vi "PercentageToRGB.vi"(10 "percentage":dbl(slide) scale=0.0..1.0) -> (2 "rgb":u32)   [LabVIEW 2017]
panel:
  out "Array":dbl[](array[numeric])
  out "log(x)":dbl[](array[numeric])
  out "Color Box":u32(colorbox)
  in  "type":enum16{"Temperature", "Greyscale", "Heatmap"}(ring)=enum."Heatmap"
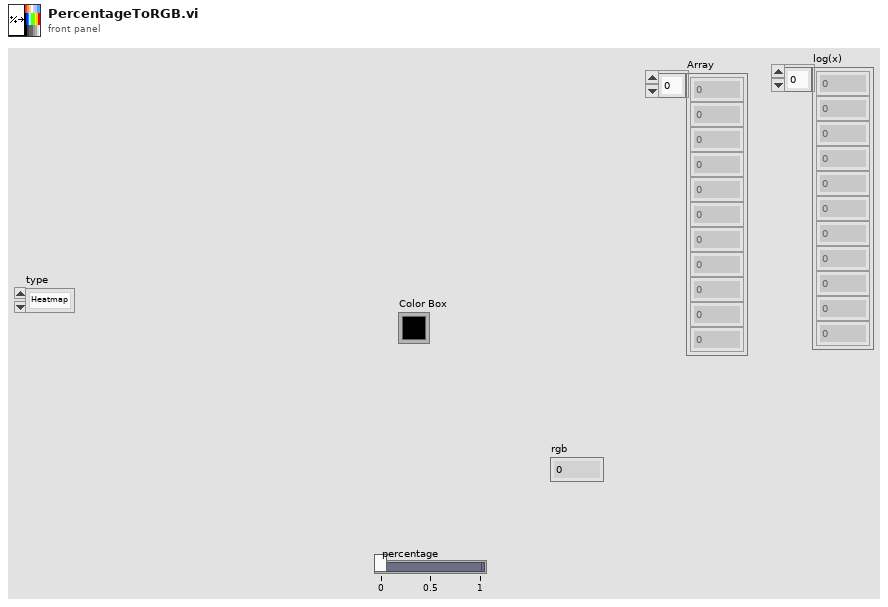
[diagram p1: front panel]
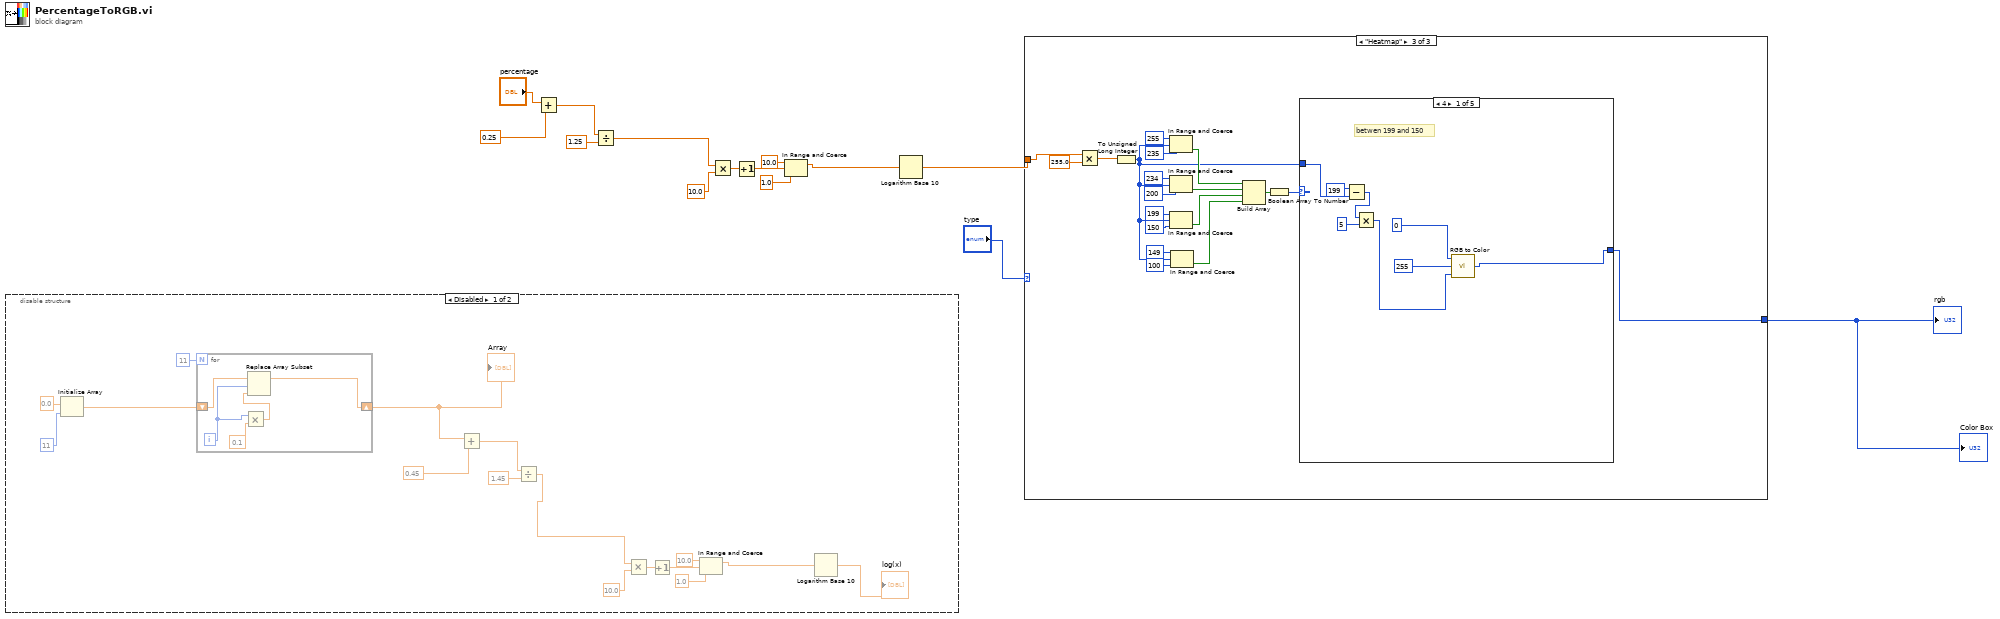
[diagram p0: block diagram]
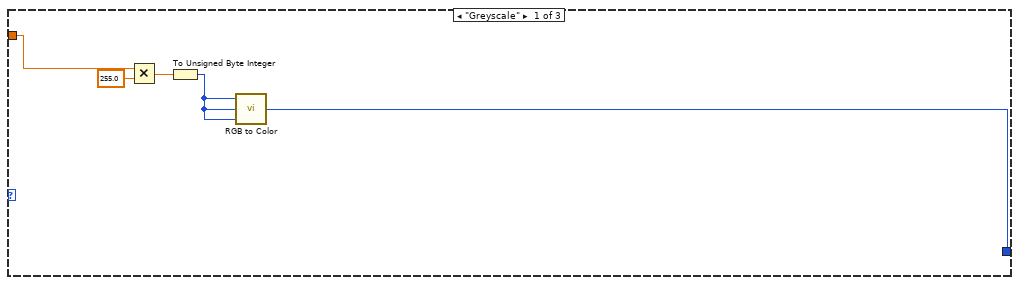
[diagram p3: hidden frame]
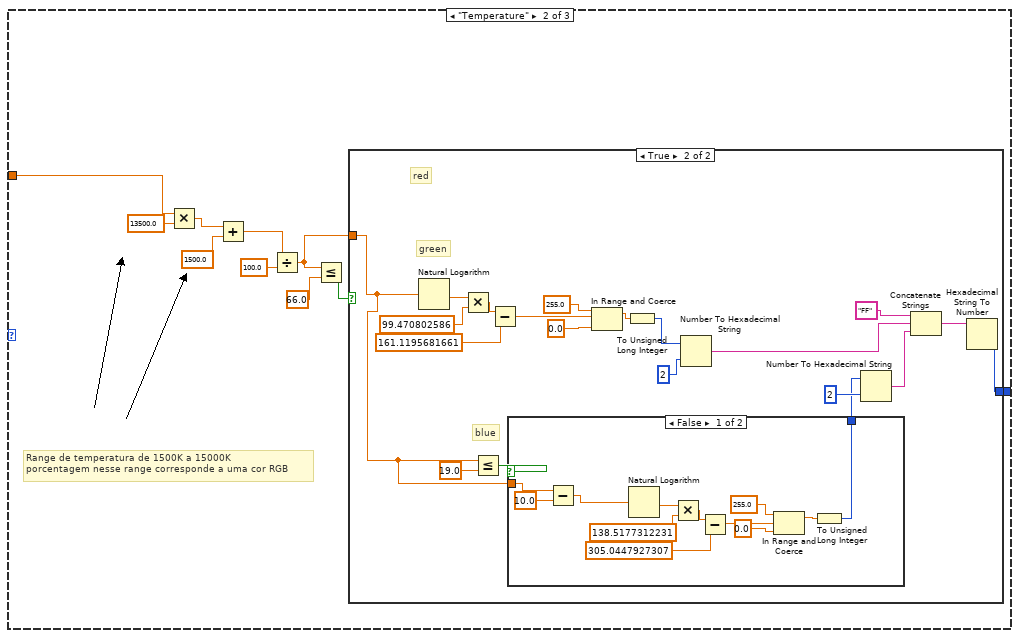
[diagram p4: hidden frame]
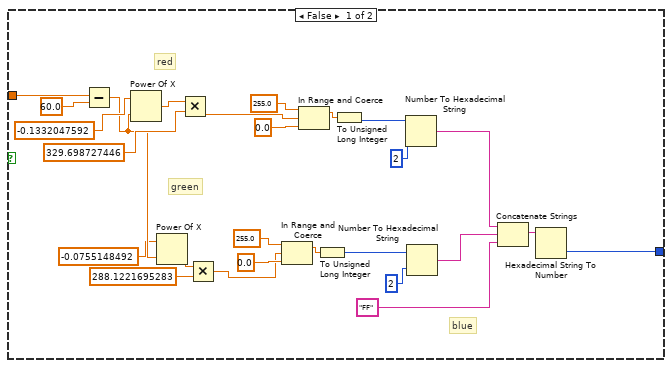
[diagram p5: hidden frame]
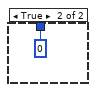
[diagram p6: hidden frame]
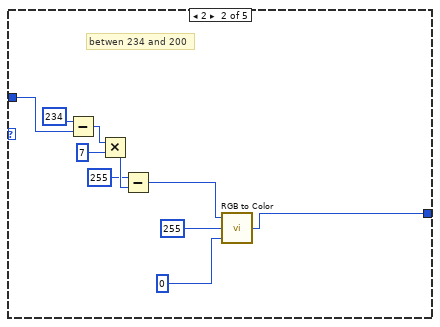
[diagram p7: hidden frame]
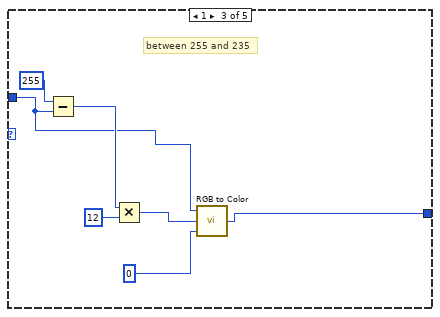
[diagram p8: hidden frame]
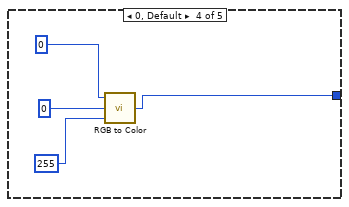
[diagram p9: hidden frame]
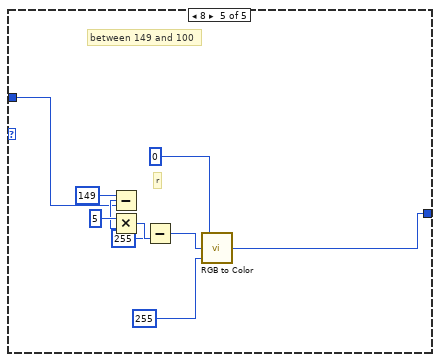
[diagram p10: hidden frame]
diagram:
  n1 = disable-structure shown="Disabled" {
    frame Disabled {
      n2 = Initialize Array(0.0 ("element"), 11 ("dimension size")) -> (w29:dbl[])
      n3 = for {
        N: 11 -> [_]
        shift-right: [w31] -> w16
        shift-left: w29 -> [w35]
        i -> [w33]
        n4 = Multiply(x=w33, y=0.1) -> (x*y=w34:dbl)
        n5 = Replace Array Subset(array=w35, new element=w34, index=w33) -> (w31:dbl[])
      }
      "Array" <- w16
      n6 = Add(x=w16, y=0.45) -> (x+y=w18:dbl[])
      n7 = Divide(x=w18, y=1.45) -> (x/y=w15:dbl[])
      n8 = Multiply(x=w15, y=10.0) -> (x*y=w25:dbl[])
      n9 = Increment(x=w25) -> (x+1=w24:dbl[])
      n10 = In Range and Coerce(upper limit=10.0, x=w24, lower limit=1.0) -> (coerced(x)=w21:dbl[])  [unwired: 1 out]
      n11 = Logarithm Base 10(1:w21) -> (0:→"log(x)":dbl[])
    }
    frame Enabled {
    }
  }
  n12 = Add(x="percentage", y=0.25) -> (x+y=w3:dbl)
  n13 = Divide(x=w3, y=1.25) -> (x/y=w1:dbl)
  n14 = Multiply(x=w1, y=10.0) -> (x*y=w11:dbl)
  n15 = Increment(x=w11) -> (x+1=w9:dbl)
  n16 = In Range and Coerce(upper limit=10.0, x=w9, lower limit=1.0) -> (coerced(x)=w6:dbl)  [unwired: 1 out]
  n17 = Logarithm Base 10(1:w6) -> (0:w10:dbl)
  n18 = case shown="\"Heatmap\"" "type" {
    tunnel: w10 -> [w40 w48 w128]
    tunnel: [w36 w43 w110] -> w13
    frame "Greyscale" {
      n19 = Multiply(x=w40, y=255.0) -> (x*y=w38:dbl)
      n20 = To Unsigned Byte Integer(number=w38) -> (unsigned 8bit integer=w37:u8)
      n21 = call <vilib>:"RGB to Color.vi"("B"=w37, "G"=w37, "R"=w37) -> ("Color"=w36:u32)
    }
    frame "Temperature" {
      # "Range de temperatura de 1500K a 15000K\nporcentagem nesse range corresponde a uma cor RGB"
      n22 = Multiply(x=w48, y=13500.0) -> (x*y=w49:dbl)
      n23 = Add(x=w49, y=1500.0) -> (x+y=w41:dbl)
      n24 = Divide(x=w41, y=100.0) -> (x/y=w44:dbl)
      n25 = Less Or Equal?(x=w44, y=66.0) -> (x <= y?=w45:bool)
      n26 = case shown="True" w45 {
        tunnel: w44 -> [w76 w85]
        tunnel: [w64 w88] -> w43
        frame False {
          # "blue"
          # "green"
          # "red"
          n27 = Subtract(x=w76, y=60.0) -> (x-y=w52:dbl)
          n28 = Power Of X(1:w52, 2:-0.1332047592 ("x")) -> (0:w74:dbl)
          n29 = Power Of X(1:w52, 2:-0.0755148492 ("x")) -> (0:w72:dbl)
          n30 = Multiply(x=w74, y=329.698727446) -> (x*y=w60:dbl)
          n31 = Multiply(x=w72, y=288.1221695283) -> (x*y=w55:dbl)
          n32 = In Range and Coerce(upper limit=255.0, x=w55, lower limit=0.0) -> (coerced(x)=w56:dbl)  [unwired: 1 out]
          n33 = In Range and Coerce(upper limit=255.0, x=w60, lower limit=0.0) -> (coerced(x)=w61:dbl)  [unwired: 1 out]
          n34 = To Unsigned Long Integer(number=w56) -> (unsigned 32bit integer=w54:u32)
          n35 = To Unsigned Long Integer(number=w61) -> (unsigned 32bit integer=w59:u32)
          n36 = Number To Hexadecimal String(1:i16 2 ("width (-)"), 2:w59) -> (0:w68:string)
          n37 = Number To Hexadecimal String(1:i16 2 ("width (-)"), 2:w54) -> (0:w67:string)
          n38 = Concatenate Strings(w68, w67, "FF" ("string")) -> (w65:string)
          n39 = Hexadecimal String To Number(string=w65) -> (number=w64:u32)  [unwired: 2 in, 1 out]
        }
        frame True {
          # "blue"
          # "green"
          # "red"
          n40 = Natural Logarithm(1:w85) -> (0:w95:dbl)
          n41 = Multiply(x=w95, y=99.470802586) -> (x*y=w93:dbl)
          n42 = Less Or Equal?(x=w85, y=19.0) -> (x <= y?=w86:bool)
          n43 = Subtract(x=w93, y=161.1195681661) -> (x-y=w84:dbl)
          n44 = case shown="False" w86 {
            tunnel: w85 -> [w104 _]
            tunnel: [w97 u32 0] -> w78
            frame False {
              n45 = Subtract(x=w104, y=10.0) -> (x-y=w102:dbl)
              n46 = Natural Logarithm(1:w102) -> (0:w108:dbl)
              n47 = Multiply(x=w108, y=138.5177312231) -> (x*y=w106:dbl)
              n48 = Subtract(x=w106, y=305.0447927307) -> (x-y=w98:dbl)
              n49 = In Range and Coerce(upper limit=255.0, x=w98, lower limit=0.0) -> (coerced(x)=w99:dbl)  [unwired: 1 out]
              n50 = To Unsigned Long Integer(number=w99) -> (unsigned 32bit integer=w97:u32)
            }
            frame True {
            }
          }
          n51 = In Range and Coerce(upper limit=255.0, x=w84, lower limit=0.0) -> (coerced(x)=w81:dbl)  [unwired: 1 out]
          n52 = To Unsigned Long Integer(number=w81) -> (unsigned 32bit integer=w80:u32)
          n53 = Number To Hexadecimal String(1:i16 2 ("width (-)"), 2:w80) -> (0:w90:string)
          n54 = Number To Hexadecimal String(1:i16 2 ("width (-)"), 2:w78) -> (0:w77:string)
          n55 = Concatenate Strings("FF", w90, w77) -> (w89:string)
          n56 = Hexadecimal String To Number(string=w89) -> (number=w88:u32)  [unwired: 2 in, 1 out]
        }
      }
    }
    frame "Heatmap" {
      n57 = Multiply(x=w128, y=255.0) -> (x*y=w126:dbl)
      n58 = To Unsigned Long Integer(number=w126) -> (unsigned 32bit integer=w111:u32)
      n59 = In Range and Coerce(upper limit=u32 234, x=w111, lower limit=u32 200) -> (In Range?=w116:bool)  [unwired: 1 out]
      n60 = In Range and Coerce(upper limit=u32 255, x=w111, lower limit=u32 235) -> (In Range?=w117:bool)  [unwired: 1 out]
      n61 = In Range and Coerce(upper limit=u32 199, x=w111, lower limit=u32 150) -> (In Range?=w115:bool)  [unwired: 1 out]
      n62 = In Range and Coerce(upper limit=u32 149, x=w111, lower limit=u32 100) -> (In Range?=w114:bool)  [unwired: 1 out]
      n63 = Build Array(w117, w116, w115, w114) -> (w113:bool[])
      n64 = Boolean Array To Number(Boolean array=w113) -> (number=w112:u32)
      n65 = case shown="4" w112 {
        tunnel: w111 -> [w136 w146 w150 _ w164]
        tunnel: [w129 w137 w147 w154 w158] -> w110
        frame 4 {
          # "betwen 199 and 150"
          n66 = Subtract(x=u32 199, y=w136) -> (x-y=w134:u32)
          n67 = Multiply(x=w134, y=u32 5) -> (x*y=w132:u32)
          n68 = call <vilib>:"RGB to Color.vi"("B"=w132, "G"=255 ("number"), "R"=0) -> ("Color"=w129:u32)
        }
        frame 2 {
          # "betwen 234 and 200"
          n69 = Subtract(x=u32 234, y=w146) -> (x-y=w144:u32)
          n70 = Multiply(x=w144, y=u32 7) -> (x*y=w142:u32)
          n71 = Subtract(x=u32 255, y=w142) -> (x-y=w138:u32)
          n72 = call <vilib>:"RGB to Color.vi"("B"=0, "G"=255, "R"=w138) -> ("Color"=w137:u32)
        }
        frame 1 {
          # "between 255 and 235"
          n73 = Subtract(x=u32 255, y=w150) -> (x-y=w152:u32)
          n74 = Multiply(x=w152, y=u32 12) -> (x*y=w149:u32)
          n75 = call <vilib>:"RGB to Color.vi"("B"=0, "G"=w149, "R"=w150) -> ("Color"=w147:u32)
        }
        frame 0, Default {
          n76 = call <vilib>:"RGB to Color.vi"("B"=255, "G"=0, "R"=0) -> ("Color"=w154:u32)
        }
        frame 8 {
          # "r"
          # "between 149 and 100"
          n77 = Subtract(x=u32 149, y=w164) -> (x-y=w165:u32)
          n78 = Multiply(x=u32 5, y=w165) -> (x*y=w163:u32)
          n79 = Subtract(x=u32 255, y=w163) -> (x-y=w160:u32)
          n80 = call <vilib>:"RGB to Color.vi"("B"=255, "G"=w160, "R"=0 ("number")) -> ("Color"=w158:u32)
        }
      }
    }
  }
  "rgb" <- w13
  "Color Box" <- w13
